vi "BRig_RT_panel_Laser1_v1,18.vi"(7 "input_setValues":bool, 9 "input_dataExp":u16[](array[numeric]), 11 "input_dataLC":u16[](array[numeric])) -> (1 "output_dataExp":u16[](array[numeric]), 3 "output_dataLC":u16[](array[numeric]))   [LabVIEW 2014]
panel:
  in  "LC_Wro_nRew2":u16
  in  "LC_Wro_nRew1":u16
  in  "LC_Rew_nRew2":u16
  in  "LC_Rew_nRew1":u16
  in  "LC_Sel_nRew2":u16
  in  "LC_Sel_nRew1":u16
  in  "LC_Cue_nRew2":u16
  in  "LC_Cue_nRew1":u16
  in  "LC_ENL_nRew2":u16
  in  "LC_ENL_nRew1":u16
  out "LaserPulseTrain":cluster{u16[], u16[]}(graph)
  in  "LED_baseline":bool
  in  "Laser_power_step":dbl
  in  "Laser_power_max":dbl
  in  "Laser_power_min":dbl
  in  "Laser_Tshutter":u16=2
  in  "Laser_Freq":u16=10
  in  "Laser_Tpeak":u16=2
  in  "Laser_T":u16
  in  "LC_Sel_PostR_Count":u16
  in  "LC_Sel_PostR_Probability":u16
  in  "LC_Sel_PostR_Block":u16(slide) max=2 step=1 scale=0.0..2.0
  in  "LC_Sel_PostR_OnOff":bool
  in  "LC_Sel_PostR_Tdelay":u16
  in  "LC_Cue_PostR_Count":u16
  in  "LC_Cue_PostR_delayOpt":bool
  in  "LC_Cue_PostR_Probability":u16
  in  "LC_Cue_PostR_Block":u16(slide) max=2 step=1 scale=0.0..2.0
  in  "LC_Cue_PostR_OnOff":bool
  in  "LC_Cue_PostR_Tdelay":u16
  in  "LC_ENL_PostR_delayOpt":bool
  in  "LC_ENL_PostR_Count":u16
  in  "LC_ENL_PostR_Probability":u16 max=100 step=1
  in  "LC_ENL_PostR_Block":u16(slide) max=2 step=1 scale=0.0..2.0
  in  "LC_ENL_PostR_OnOff":bool
  in  "LC_ENL_PostR_Tdelay":u16
  in  "LC_Sel_PreR_Count":u16
  in  "LC_Sel_First_Count":u16
  in  "LC_Sel_PreR_Probability":u16
  in  "LC_Sel_PreR_Block":u16(slide) max=2 step=1 scale=0.0..2.0
  in  "LC_Sel_PreR_OnOff":bool
  in  "LC_Sel_First_Probability":u16
  in  "LC_Sel_First_Block":u16(slide) max=2 step=1 scale=0.0..2.0
  in  "LC_Sel_First_OnOff":bool
  in  "LC_Sel_PreR_Tdelay":u16
  in  "LC_Sel_First_Tdelay":u16
  in  "LC_Cue_PreR_Count":u16
  in  "LC_Cue_First_Count":u16
  in  "LC_Cue_PreR_delayOpt":bool
  in  "LC_ENL_PreR_delayOpt":bool
  in  "LC_ENL_PreR_Count":u16
  in  "LC_ENL_First_Count":u16
  in  "LC_Cue_First_delayOpt":bool
  in  "LC_ENL_First_delayOpt":bool
  in  "LC_Wrong_Probability":u16
  in  "LC_Wrong_Trial":u16(slide) max=4 step=1 scale=0.0..4.0
  in  "LC_Wrong_Block":u16(slide) max=2 step=1 scale=0.0..2.0
  in  "LC_Wrong_OnOff":bool
  in  "LC_Reward_Probability":u16
  in  "LC_Reward_Trial":u16(slide) max=3 step=1 scale=0.0..3.0
  in  "LC_Reward_Block":u16(slide) max=2 step=1 scale=0.0..2.0
  in  "LC_Reward_OnOff":bool
  in  "LC_Cue_PreR_Probability":u16
  in  "LC_Cue_PreR_Block":u16(slide) max=2 step=1 scale=0.0..2.0
  in  "LC_Cue_PreR_OnOff":bool
  in  "LC_Cue_First_Probability":u16
  in  "LC_Cue_First_Block":u16(slide) max=2 step=1 scale=0.0..2.0
  in  "LC_Cue_First_OnOff":bool
  in  "LC_ENL_PreR_Probability":u16 max=100 step=1
  in  "LC_ENL_PreR_Block":u16(slide) max=2 step=1 scale=0.0..2.0
  in  "LC_ENL_PreR_OnOff":bool
  in  "LC_ENL_First_Probability":u16 max=100 step=1
  in  "LC_ENL_First_Block":u16(slide) max=2 step=1 scale=0.0..2.0
  in  "LC_Wrong_Tdelay":u16
  in  "LC_Cue_PreR_Tdelay":u16
  in  "LC_ENL_PreR_Tdelay":u16
  in  "LC_Reward_Tdelay":u16
  in  "LC_Cue_First_Tdelay":u16
  in  "LC_ENL_First_Tdelay":u16
  in  "LC_ENL_First_OnOff":bool
  # "Laser1 Control\n                               On/Off      Block        Probability [%]   Delay [ms]                              Count"
  # "Enforced\nNonLick"
  # "from end"
  # "First\nTrial"
  # "from start"
  # "from end"
  # "PreReward\nTrials"
  # "from start"
  # "from end"
  # "PostReward\nTrials"
  # "from start"
  # "PostReward Option - Trigger after [X1] or [X2] reward\n                                        (0 = ignore this option)"
  # "Cue"
  # "from end"
  # "First\nTrial"
  # "from start"
  # "from end"
  # "PreReward\nTrials"
  # "from start"
  # "from end"
  # "PostReward\nTrials"
  # "from start"
  # "PostReward Option - Trigger after [X1] or [X2] reward\n                                        (0 = ignore this option)"
  # "Selection"
  # "from start"
  # "First\nTrial"
  # "from start"
  # "PreReward\nTrials"
  # "from start"
  # "PostReward\nTrials"
  # "PostReward Option - Trigger after [X1] or [X2] reward\n                                        (0 = ignore this option)"
  # "Laser1 Parameters"
  # "Laser1 Response\n           On/Off      Block           Trial     Probability %  Delay [ms]"
  # "Frequency\n[Hz]"
  # "Selection\nReward"
  # "Timing [ms]\n Duration     Peak Width   Shutter"
  # "Trigger after [X1] or [X2] reward\n(0 = ignore this option)"
  # "Laser Power [V]\nMin          Max              Step"
  # "Selection\nWrong"
  # "Trigger after [X1] or [X2] reward\n(0 = ignore this option)"
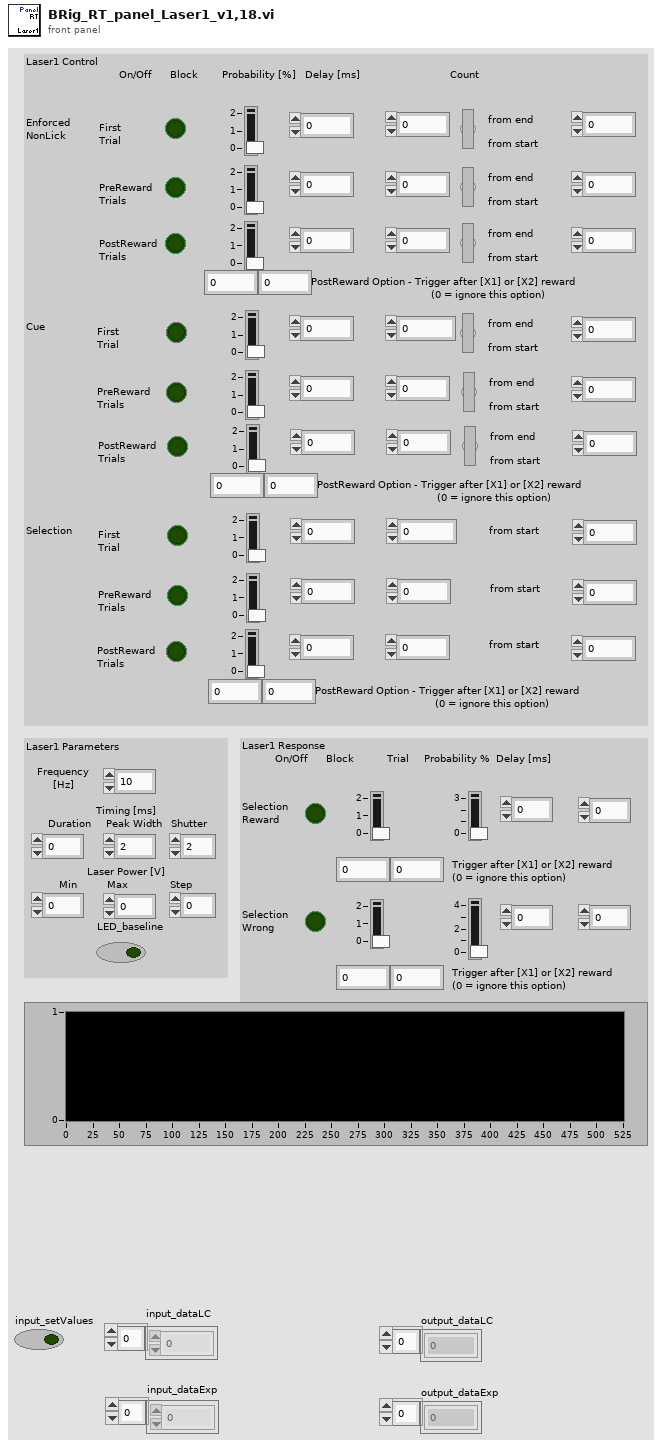
[diagram p1: front panel]
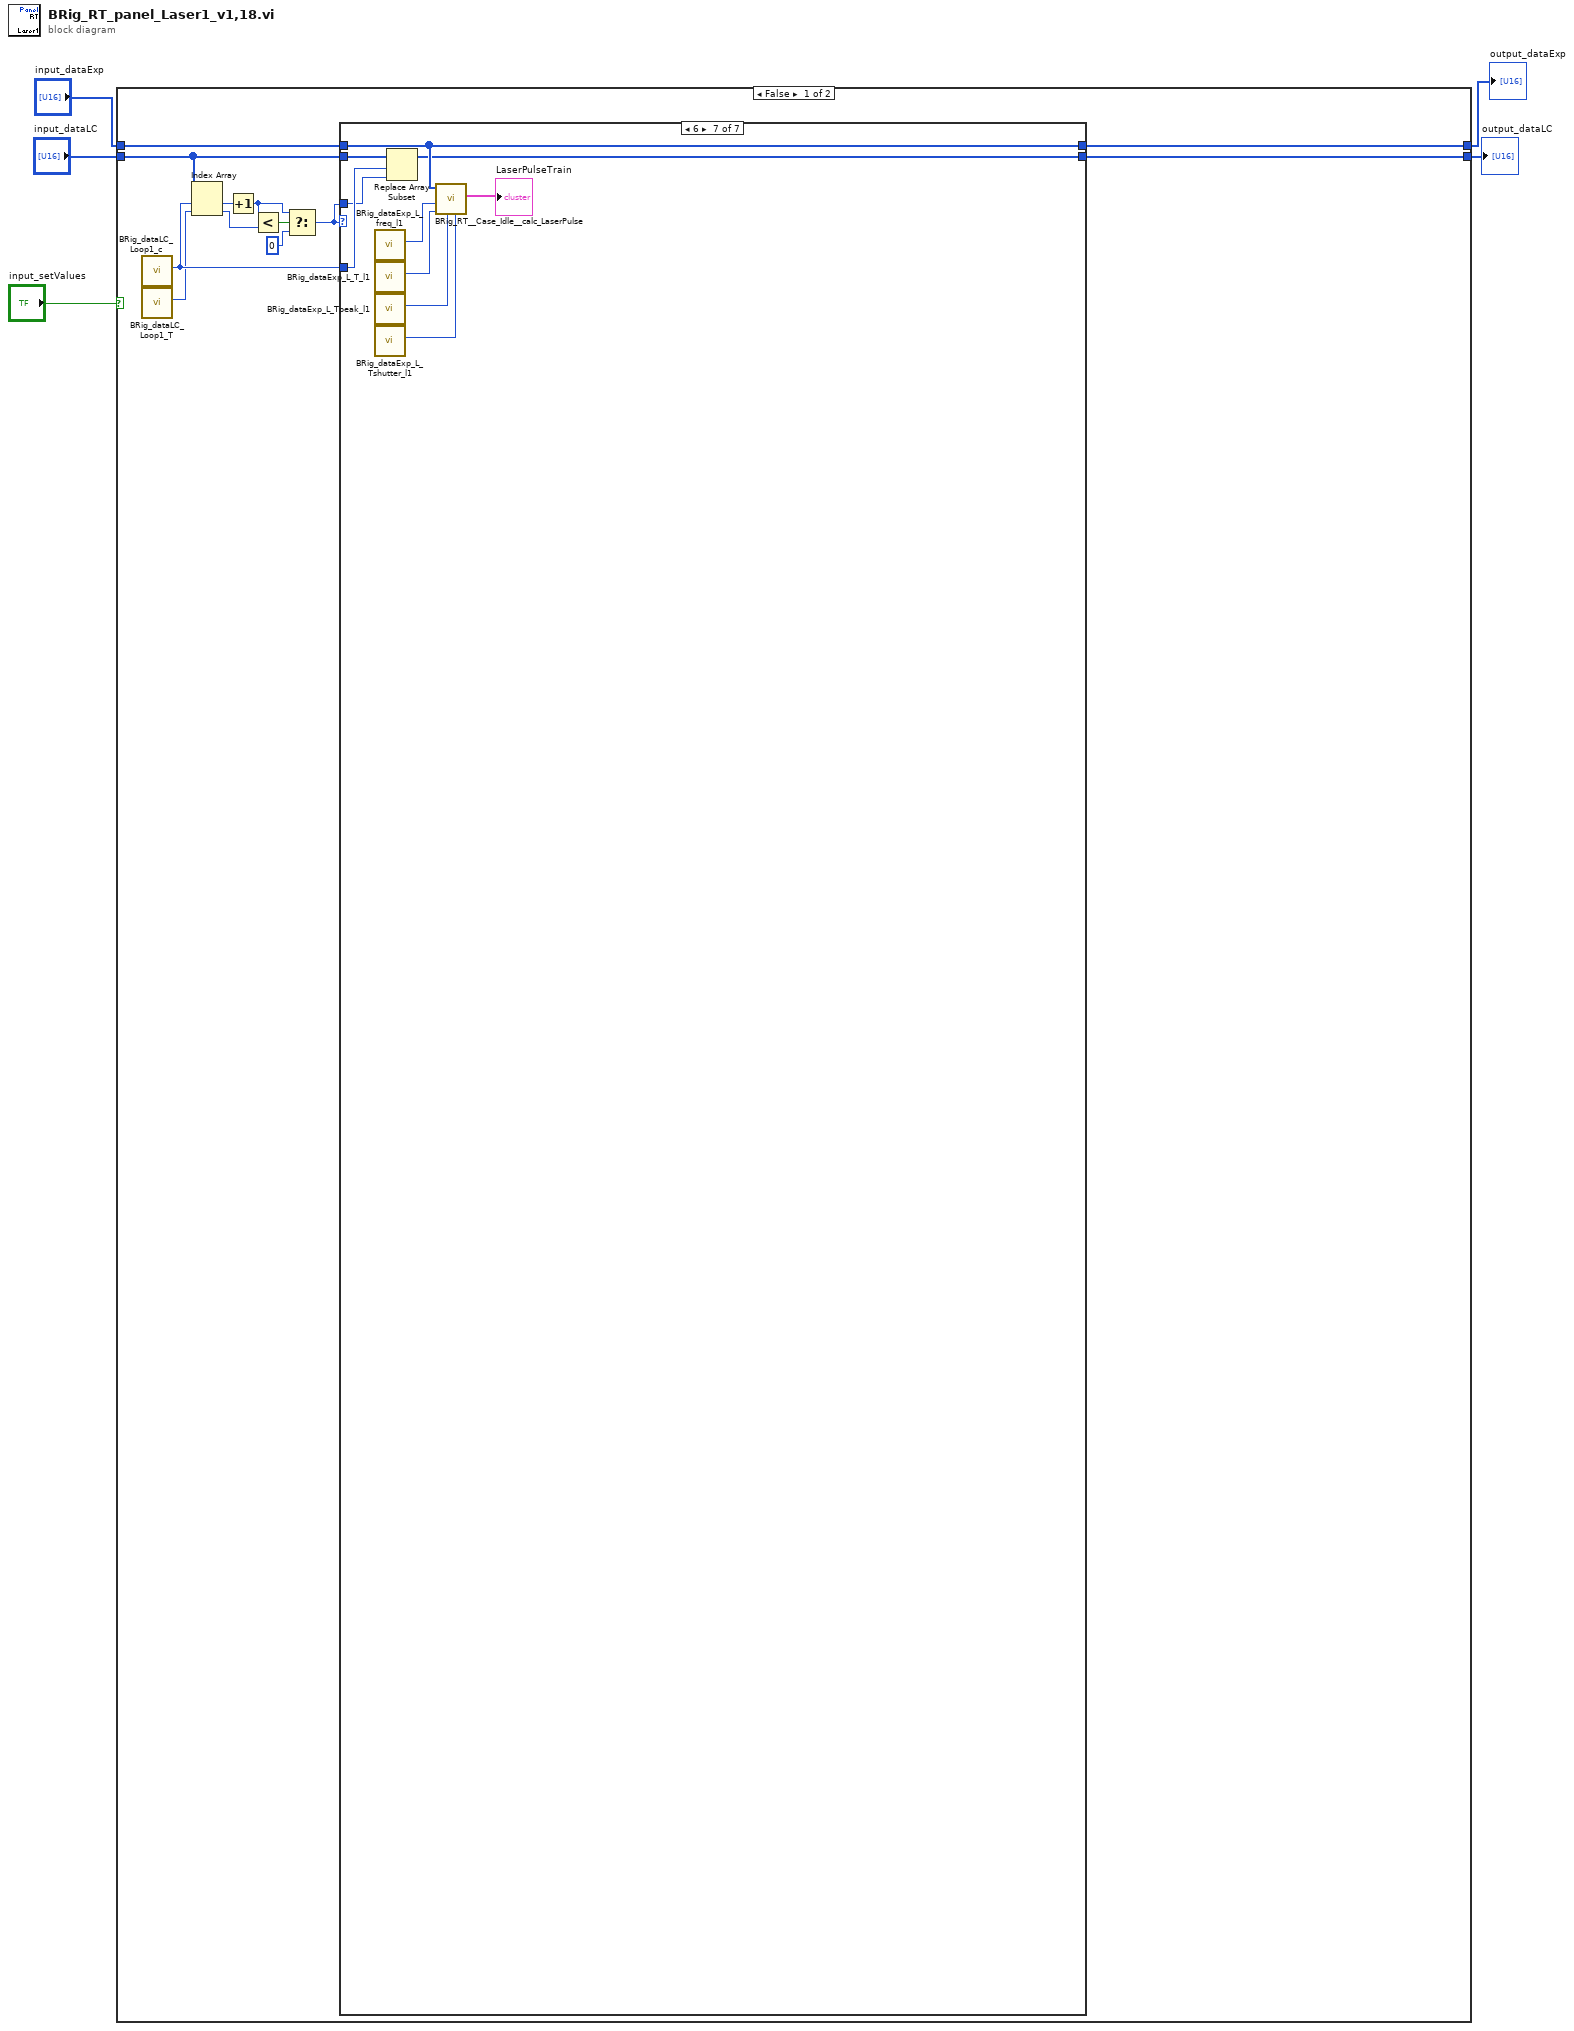
[diagram p0: block diagram]
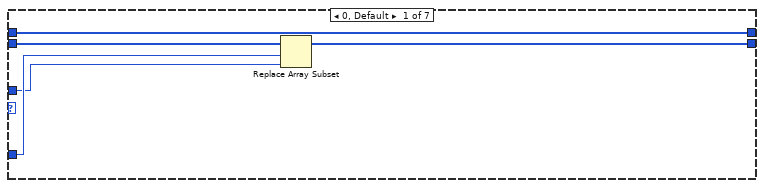
[diagram p2: hidden frame]
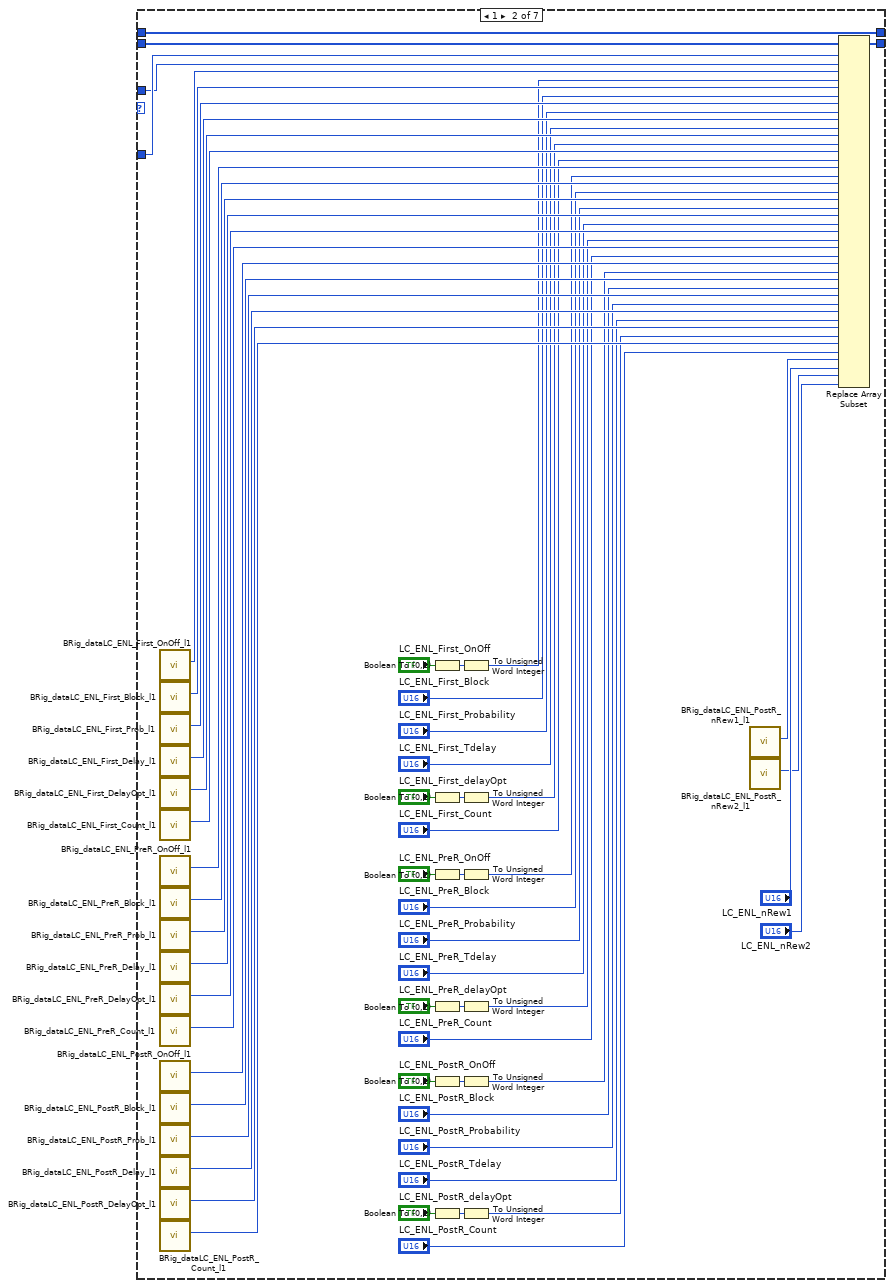
[diagram p3: hidden frame]
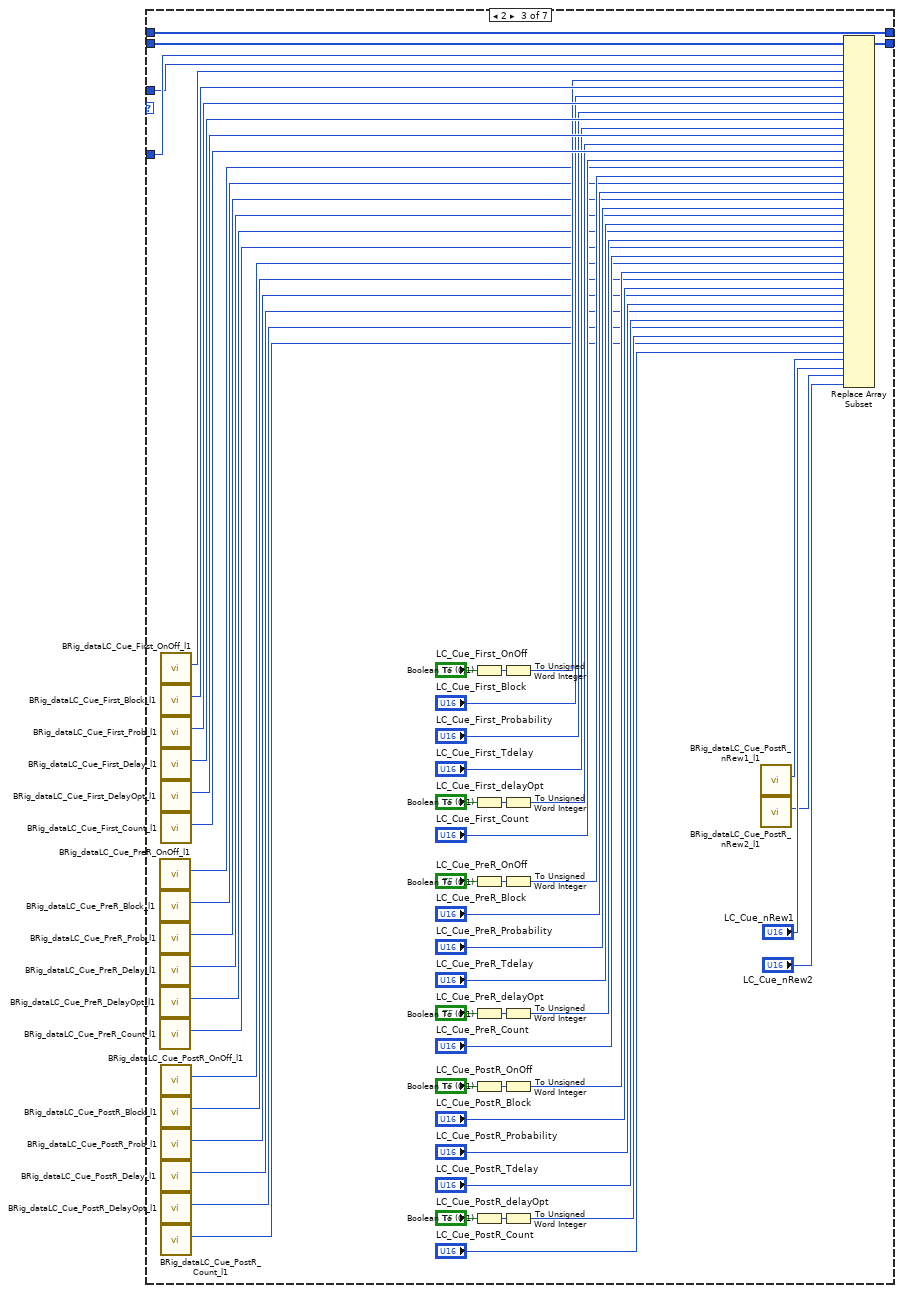
[diagram p4: hidden frame]
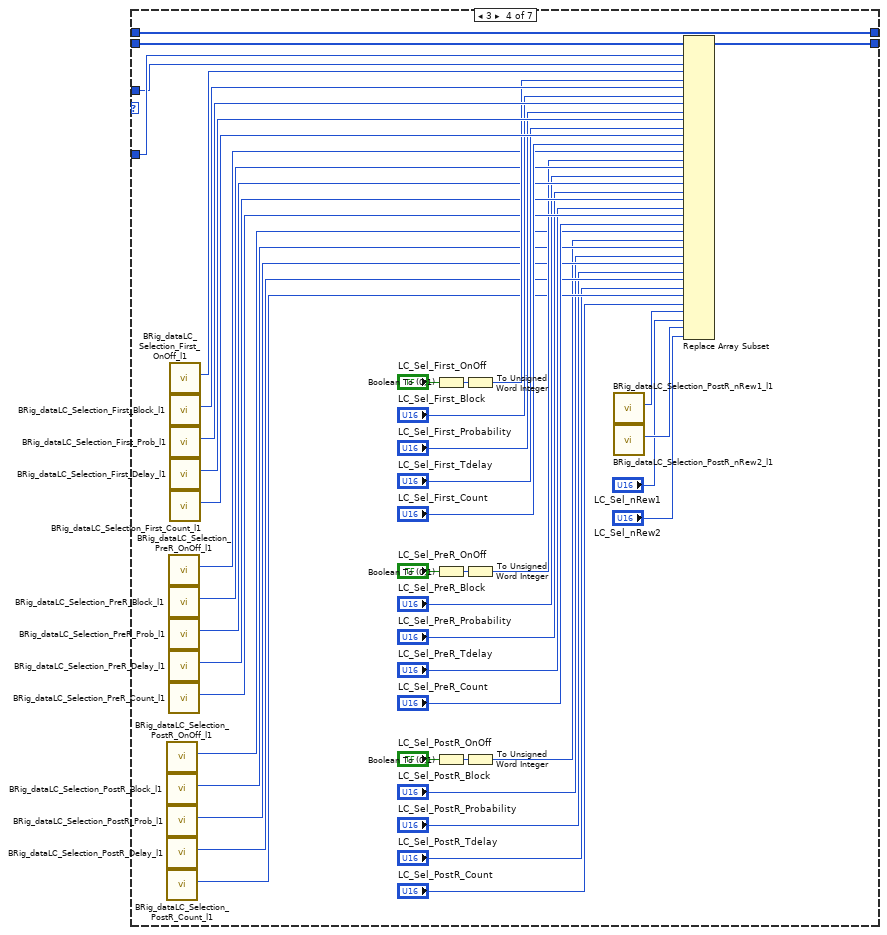
[diagram p5: hidden frame]
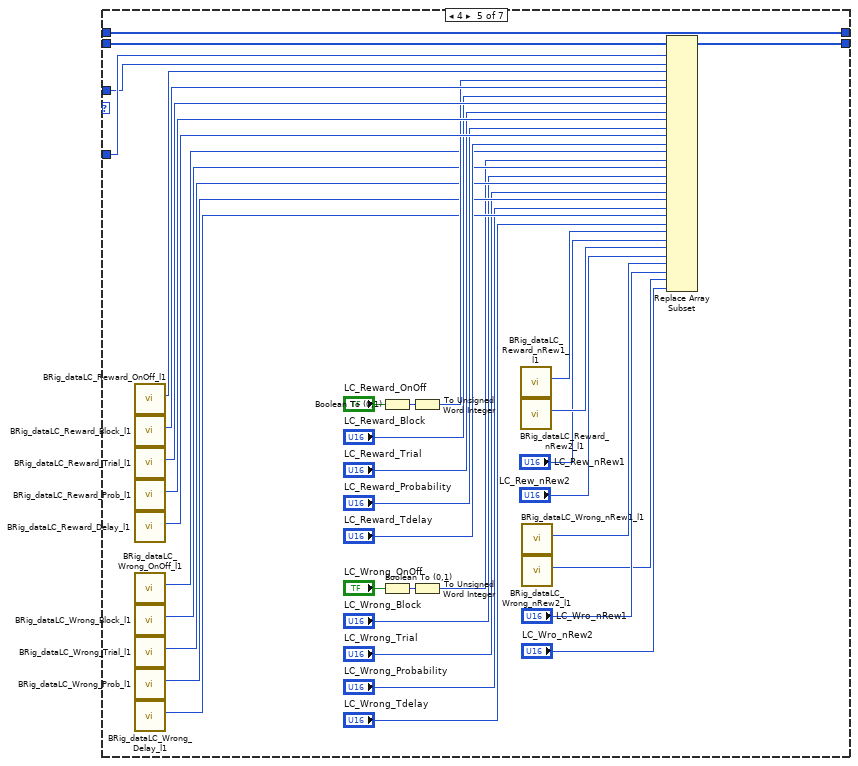
[diagram p6: hidden frame]
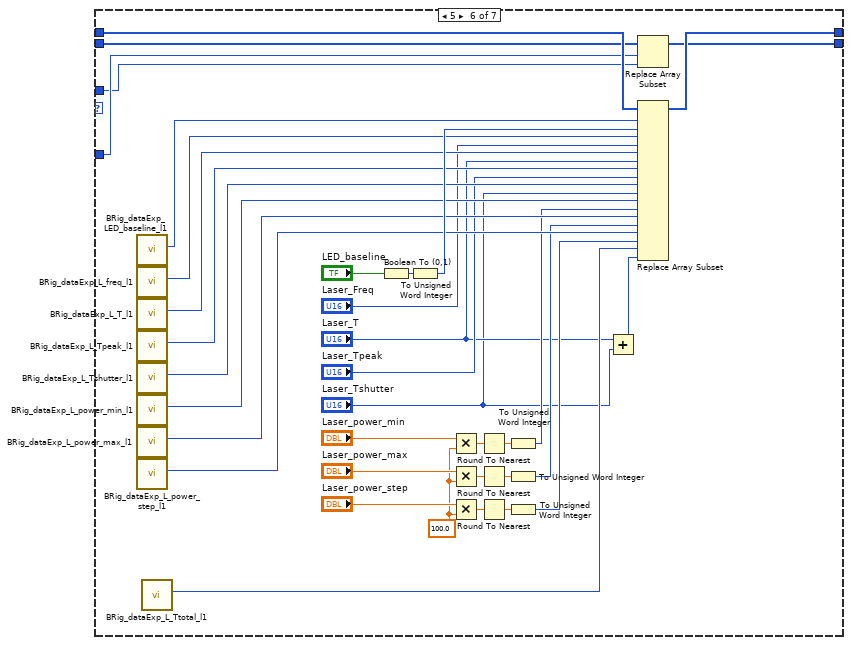
[diagram p7: hidden frame]
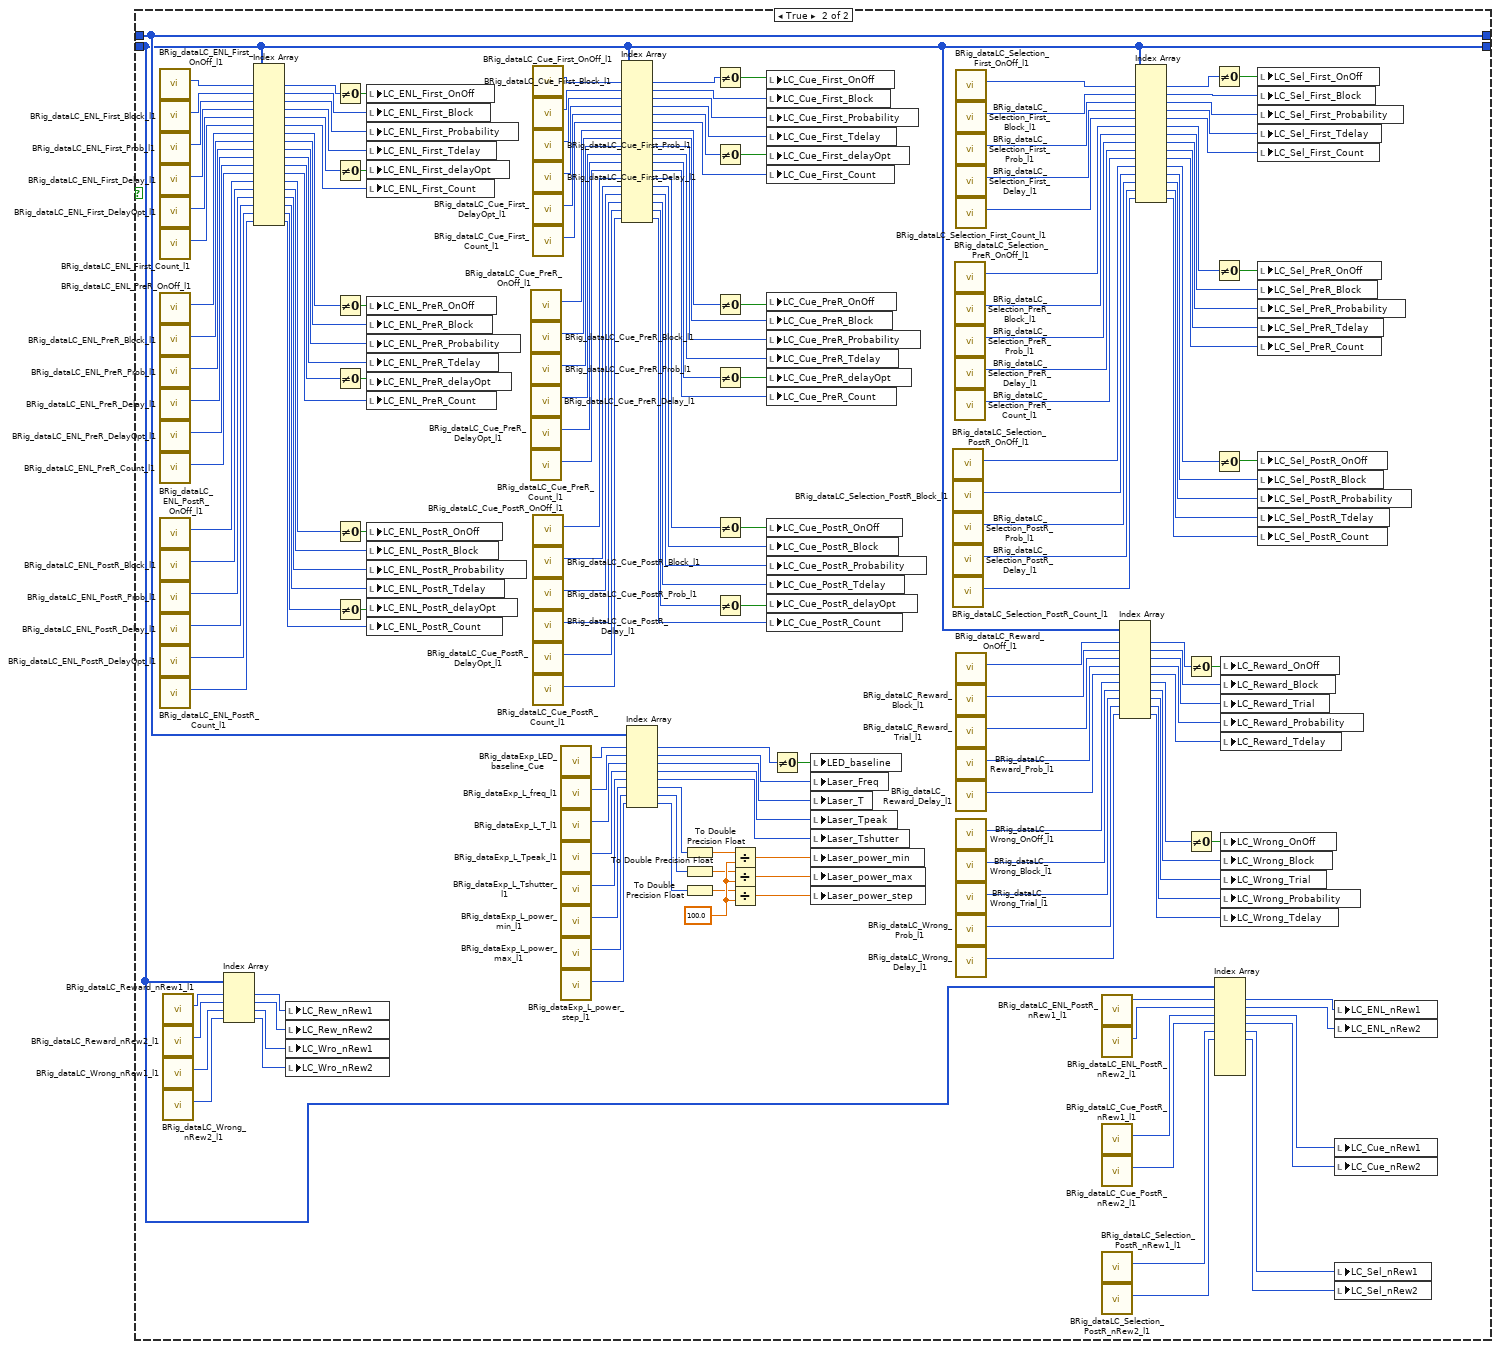
[diagram p8: hidden frame]
diagram:
  n1 = case shown="False" "input_setValues" {
    tunnel: "input_dataLC" -> [w17 w281]
    tunnel: [w11 w281] -> w4
    tunnel: "input_dataExp" -> [w7 w282]
    tunnel: [w6 w282] -> w1
    frame False {
      n2 = call "BRig_dataLC_Loop1_c.vi"() -> ("output_Loop1_c"=w10:i32)  [unwired: 11 in]
      n3 = call "BRig_dataLC_Loop1_T.vi"() -> ("output_Loop1_T"=w9:i32)  [unwired: 11 in]
      n4 = Index Array(array=w17, index #1=w10, index #2=w9) -> (element #1=w16:u16, element #2=w15:u16)
      n5 = Increment(x=w16) -> (x+1=w12:u16)
      n6 = Less?(x=w12, y=w15) -> (x < y?=w14:bool)
      n7 = Select(t=w12, s=w14, f=u16 0) -> (s? t:f=w8:u16)
      n8 = case shown="6" w8 {
        tunnel: w17 -> [w22 w79 w136 w181 w218 w223 w262]
        tunnel: w10 -> [w20 w29 w98 w143 w192 w221 w260]
        tunnel: w8 -> [w19 w28 w97 w142 w191 w220 w259]
        tunnel: [w21 w72 w135 w180 w217 w222 w261] -> w11
        tunnel: w7 -> [w18 w27 w84 w141 w190 w225 w264]
        tunnel: [w18 w27 w84 w141 w190 w224 w264] -> w6
        frame 0, Default {
          n9 = Replace Array Subset(array=w22, new element=w19, index=w20) -> (w21:u16[])
        }
        frame 1 {
          n10 = call "BRig_dataLC_ENL_First_OnOff_l1.vi"() -> ("output_ENL_First_OnOff"=w78:i32)  [unwired: 11 in]
          n11 = call "BRig_dataLC_ENL_First_Block_l1.vi"() -> ("output_ENL_First_Block"=w77:i32)  [unwired: 11 in]
          n12 = call "BRig_dataLC_ENL_First_Prob_l1.vi"() -> ("output_ENL_First_Prob"=w76:i32)  [unwired: 11 in]
          n13 = call "BRig_dataLC_ENL_First_Delay_l1.vi"() -> ("output_ENL_First_Delay"=w75:i32)  [unwired: 11 in]
          n14 = call "BRig_dataLC_ENL_First_DelayOpt_l1.vi"() -> ("output_ENL_First_DelayOpt"=w74:i32)  [unwired: 11 in]
          n15 = call "BRig_dataLC_ENL_First_Count_l1.vi"() -> ("output_ENL_First_Count"=w73:i32)  [unwired: 11 in]
          n16 = call "BRig_dataLC_ENL_PreR_OnOff_l1.vi"() -> ("output_ENL_PreR_OnOff"=w71:i32)  [unwired: 11 in]
          n17 = call "BRig_dataLC_ENL_PreR_Block_l1.vi"() -> ("output_ENL_PreR_Block"=w70:i32)  [unwired: 11 in]
          n18 = call "BRig_dataLC_ENL_PreR_Prob_l1.vi"() -> ("output_ENL_PreR_Prob"=w69:i32)  [unwired: 11 in]
          n19 = call "BRig_dataLC_ENL_PreR_Delay_l1.vi"() -> ("output_ENL_PreR_Delay"=w68:i32)  [unwired: 11 in]
          n20 = call "BRig_dataLC_ENL_PreR_DelayOpt_l1.vi"() -> ("output_ENL_PreR_DelayOpt"=w67:i32)  [unwired: 11 in]
          n21 = call "BRig_dataLC_ENL_PreR_Count_l1.vi"() -> ("output_ENL_PreR_Count"=w66:i32)  [unwired: 11 in]
          n22 = call "BRig_dataLC_ENL_PostR_OnOff_l1.vi"() -> ("output_ENL_PostR_OnOff"=w65:i32)  [unwired: 11 in]
          n23 = call "BRig_dataLC_ENL_PostR_Block_l1.vi"() -> ("output_ENL_PostR_Block"=w64:i32)  [unwired: 11 in]
          n24 = call "BRig_dataLC_ENL_PostR_Prob_l1.vi"() -> ("output_ENL_PostR_Prob"=w63:i32)  [unwired: 11 in]
          n25 = call "BRig_dataLC_ENL_PostR_Delay_l1.vi"() -> ("output_ENL_PostR_Delay"=w62:i32)  [unwired: 11 in]
          n26 = call "BRig_dataLC_ENL_PostR_DelayOpt_l1.vi"() -> ("output_ENL_PostR_DelayOpt"=w61:i32)  [unwired: 11 in]
          n27 = call "BRig_dataLC_ENL_PostR_Count_l1.vi"() -> ("output_ENL_PostR_Count"=w60:i32)  [unwired: 11 in]
          n28 = Boolean To (0,1)(Boolean="LC_ENL_First_OnOff") -> (0, 1=w58:i16)
          n29 = Boolean To (0,1)(Boolean="LC_ENL_First_delayOpt") -> (0, 1=w57:i16)
          n30 = Boolean To (0,1)(Boolean="LC_ENL_PreR_OnOff") -> (0, 1=w55:i16)
          n31 = Boolean To (0,1)(Boolean="LC_ENL_PreR_delayOpt") -> (0, 1=w53:i16)
          n32 = Boolean To (0,1)(Boolean="LC_ENL_PostR_OnOff") -> (0, 1=w51:i16)
          n33 = Boolean To (0,1)(Boolean="LC_ENL_PostR_delayOpt") -> (0, 1=w49:i16)
          n34 = To Unsigned Word Integer(number=w58) -> (unsigned 16bit integer=w47:u16)
          n35 = To Unsigned Word Integer(number=w57) -> (unsigned 16bit integer=w43:u16)
          n36 = To Unsigned Word Integer(number=w55) -> (unsigned 16bit integer=w41:u16)
          n37 = To Unsigned Word Integer(number=w53) -> (unsigned 16bit integer=w37:u16)
          n38 = To Unsigned Word Integer(number=w51) -> (unsigned 16bit integer=w35:u16)
          n39 = To Unsigned Word Integer(number=w49) -> (unsigned 16bit integer=w31:u16)
          n40 = call "BRig_dataLC_ENL_PostR_nRew1_l1.vi"() -> ("output_ENL_PostR_nRew1_l1"=w26:i32)  [unwired: 11 in]
          n41 = call "BRig_dataLC_ENL_PostR_nRew2_l1.vi"() -> ("output_ENL_PostR_nRew2_l1"=w24:i32)  [unwired: 11 in]
          n42 = Replace Array Subset(array=w79, new element #1=w28, index #1=w29, new element #2=w47, index #2=w78, new element #3="LC_ENL_First_Block", index #3=w77, new element #4="LC_ENL_First_Probability", index #4=w76, new element #5="LC_ENL_First_Tdelay", index #5=w75, new element #6=w43, index #6=w74, new element #7="LC_ENL_First_Count", index #7=w73, new element #8=w41, index #8=w71, new element #9="LC_ENL_PreR_Block", index #9=w70, new element #10="LC_ENL_PreR_Probability", index #10=w69, new element #11="LC_ENL_PreR_Tdelay", index #11=w68, new element #12=w37, index #12=w67, new element #13="LC_ENL_PreR_Count", index #13=w66, new element #14=w35, index #14=w65, new element #15="LC_ENL_PostR_Block", index #15=w64, new element #16="LC_ENL_PostR_Probability", index #16=w63, new element #17="LC_ENL_PostR_Tdelay", index #17=w62, new element #18=w31, index #18=w61, new element #19="LC_ENL_PostR_Count", index #19=w60, new element #20="LC_ENL_nRew1", index #20=w26, new element #21="LC_ENL_nRew2", index #21=w24) -> (w72:u16[])
        }
        frame 2 {
          n43 = call "BRig_dataLC_Cue_PreR_OnOff_l1.vi"() -> ("output_Cue_PreR_OnOff"=w94:i32)  [unwired: 11 in]
          n44 = call "BRig_dataLC_Cue_PreR_Block_l1.vi"() -> ("output_Cue_PreR_Block"=w93:i32)  [unwired: 11 in]
          n45 = call "BRig_dataLC_Cue_PreR_Prob_l1.vi"() -> ("output_Cue_PreR_Prob"=w92:i32)  [unwired: 11 in]
          n46 = call "BRig_dataLC_Cue_PreR_Delay_l1.vi"() -> ("output_Cue_PreR_Delay"=w91:i32)  [unwired: 11 in]
          n47 = call "BRig_dataLC_Cue_PreR_DelayOpt_l1.vi"() -> ("output_Cue_PreR_DelayOpt"=w90:i32)  [unwired: 11 in]
          n48 = call "BRig_dataLC_Cue_PreR_Count_l1.vi"() -> ("output_Cue_PreR_Count"=w95:i32)  [unwired: 11 in]
          n49 = call "BRig_dataLC_Cue_First_OnOff_l1.vi"() -> ("output_Cue_First_OnOff"=w134:i32)  [unwired: 11 in]
          n50 = call "BRig_dataLC_Cue_First_Block_l1.vi"() -> ("output_Cue_First_Block"=w133:i32)  [unwired: 11 in]
          n51 = call "BRig_dataLC_Cue_First_Prob_l1.vi"() -> ("output_Cue_First_Prob"=w132:i32)  [unwired: 11 in]
          n52 = call "BRig_dataLC_Cue_First_Delay_l1.vi"() -> ("output_Cue_First_Delay"=w131:i32)  [unwired: 11 in]
          n53 = call "BRig_dataLC_Cue_First_DelayOpt_l1.vi"() -> ("output_Cue_First_DelayOpt"=w130:i32)  [unwired: 11 in]
          n54 = call "BRig_dataLC_Cue_First_Count_l1.vi"() -> ("output_Cue_First_Count"=w129:i32)  [unwired: 11 in]
          n55 = call "BRig_dataLC_Cue_PostR_OnOff_l1.vi"() -> ("output_Cue_PostR_OnOff"=w96:i32)  [unwired: 11 in]
          n56 = call "BRig_dataLC_Cue_PostR_Block_l1.vi"() -> ("output_Cue_PostR_Block"=w89:i32)  [unwired: 11 in]
          n57 = call "BRig_dataLC_Cue_PostR_Prob_l1.vi"() -> ("output_Cue_PostR_Prob"=w88:i32)  [unwired: 11 in]
          n58 = call "BRig_dataLC_Cue_PostR_Delay_l1.vi"() -> ("output_Cue_PostR_Delay"=w87:i32)  [unwired: 11 in]
          n59 = call "BRig_dataLC_Cue_PostR_DelayOpt_l1.vi"() -> ("output_Cue_PostR_DelayOpt"=w86:i32)  [unwired: 11 in]
          n60 = call "BRig_dataLC_Cue_PostR_Count_l1.vi"() -> ("output_Cue_PostR_Count"=w85:i32)  [unwired: 11 in]
          n61 = Boolean To (0,1)(Boolean="LC_Cue_First_OnOff") -> (0, 1=w122:i16)
          n62 = Boolean To (0,1)(Boolean="LC_Cue_First_delayOpt") -> (0, 1=w121:i16)
          n63 = Boolean To (0,1)(Boolean="LC_Cue_PreR_OnOff") -> (0, 1=w120:i16)
          n64 = Boolean To (0,1)(Boolean="LC_Cue_PreR_delayOpt") -> (0, 1=w119:i16)
          n65 = Boolean To (0,1)(Boolean="LC_Cue_PostR_OnOff") -> (0, 1=w118:i16)
          n66 = Boolean To (0,1)(Boolean="LC_Cue_PostR_delayOpt") -> (0, 1=w117:i16)
          n67 = To Unsigned Word Integer(number=w122) -> (unsigned 16bit integer=w116:u16)
          n68 = To Unsigned Word Integer(number=w121) -> (unsigned 16bit integer=w112:u16)
          n69 = To Unsigned Word Integer(number=w120) -> (unsigned 16bit integer=w110:u16)
          n70 = To Unsigned Word Integer(number=w119) -> (unsigned 16bit integer=w106:u16)
          n71 = To Unsigned Word Integer(number=w118) -> (unsigned 16bit integer=w104:u16)
          n72 = To Unsigned Word Integer(number=w117) -> (unsigned 16bit integer=w100:u16)
          n73 = call "BRig_dataLC_Cue_PostR_nRew1_l1.vi"() -> ("output_Cue_PostR_nRew1_l1"=w83:i32)  [unwired: 11 in]
          n74 = call "BRig_dataLC_Cue_PostR_nRew2_l1.vi"() -> ("output_Cue_PostR_nRew2_l1"=w81:i32)  [unwired: 11 in]
          n75 = Replace Array Subset(array=w136, new element #1=w97, index #1=w98, new element #2=w116, index #2=w134, new element #3="LC_Cue_First_Block", index #3=w133, new element #4="LC_Cue_First_Probability", index #4=w132, new element #5="LC_Cue_First_Tdelay", index #5=w131, new element #6=w112, index #6=w130, new element #7="LC_Cue_First_Count", index #7=w129, new element #8=w110, index #8=w94, new element #9="LC_Cue_PreR_Block", index #9=w93, new element #10="LC_Cue_PreR_Probability", index #10=w92, new element #11="LC_Cue_PreR_Tdelay", index #11=w91, new element #12=w106, index #12=w90, new element #13="LC_Cue_PreR_Count", index #13=w95, new element #14=w104, index #14=w96, new element #15="LC_Cue_PostR_Block", index #15=w89, new element #16="LC_Cue_PostR_Probability", index #16=w88, new element #17="LC_Cue_PostR_Tdelay", index #17=w87, new element #18=w100, index #18=w86, new element #19="LC_Cue_PostR_Count", index #19=w85, new element #20="LC_Cue_nRew1", index #20=w83, new element #21="LC_Cue_nRew2", index #21=w81) -> (w135:u16[])
        }
        frame 3 {
          n76 = call "BRig_dataLC_Selection_PostR_OnOff_l1.vi"() -> ("output_Selection_PostR_OnOff"=w153:i32)  [unwired: 11 in]
          n77 = call "BRig_dataLC_Selection_PostR_Block_l1.vi"() -> ("output_Selection_PostR_Block"=w152:i32)  [unwired: 11 in]
          n78 = call "BRig_dataLC_Selection_PostR_Prob_l1.vi"() -> ("output_Selection_PostR_Prob"=w151:i32)  [unwired: 11 in]
          n79 = call "BRig_dataLC_Selection_PostR_Delay_l1.vi"() -> ("output_Selection_PostR_Delay"=w150:i32)  [unwired: 11 in]
          n80 = call "BRig_dataLC_Selection_PostR_Count_l1.vi"() -> ("output_Selection_PostR_Count"=w149:i32)  [unwired: 11 in]
          n81 = call "BRig_dataLC_Selection_PreR_OnOff_l1.vi"() -> ("output_Selection_PreR_OnOff"=w163:i32)  [unwired: 11 in]
          n82 = call "BRig_dataLC_Selection_PreR_Block_l1.vi"() -> ("output_Selection_PreR_Block"=w162:i32)  [unwired: 11 in]
          n83 = call "BRig_dataLC_Selection_PreR_Prob_l1.vi"() -> ("output_Selection_PreR_Prob"=w161:i32)  [unwired: 11 in]
          n84 = call "BRig_dataLC_Selection_PreR_Delay_l1.vi"() -> ("output_Selection_PreR_Delay"=w160:i32)  [unwired: 11 in]
          n85 = call "BRig_dataLC_Selection_PreR_Count_l1.vi"() -> ("output_Selection_PreR_Count"=w159:i32)  [unwired: 11 in]
          n86 = call "BRig_dataLC_Selection_First_OnOff_l1.vi"() -> ("output_Selection_First_OnOff"=w173:i32)  [unwired: 11 in]
          n87 = call "BRig_dataLC_Selection_First_Block_l1.vi"() -> ("output_Selection_First_Block"=w172:i32)  [unwired: 11 in]
          n88 = call "BRig_dataLC_Selection_First_Prob_l1.vi"() -> ("output_Selection_First_Prob"=w171:i32)  [unwired: 11 in]
          n89 = call "BRig_dataLC_Selection_First_Delay_l1.vi"() -> ("output_Selection_First_Delay"=w170:i32)  [unwired: 11 in]
          n90 = call "BRig_dataLC_Selection_First_Count_l1.vi"() -> ("output_Selection_First_Count"=w169:i32)  [unwired: 11 in]
          n91 = Boolean To (0,1)(Boolean="LC_Sel_First_OnOff") -> (0, 1=w176:i16)
          n92 = Boolean To (0,1)(Boolean="LC_Sel_PreR_OnOff") -> (0, 1=w175:i16)
          n93 = Boolean To (0,1)(Boolean="LC_Sel_PostR_OnOff") -> (0, 1=w174:i16)
          n94 = To Unsigned Word Integer(number=w176) -> (unsigned 16bit integer=w168:u16)
          n95 = To Unsigned Word Integer(number=w175) -> (unsigned 16bit integer=w158:u16)
          n96 = To Unsigned Word Integer(number=w174) -> (unsigned 16bit integer=w148:u16)
          n97 = call "BRig_dataLC_Selection_PostR_nRew1_l1.vi"() -> ("output_Selection_PostR_nRew1_l1"=w140:i32)  [unwired: 11 in]
          n98 = call "BRig_dataLC_Selection_PostR_nRew2_l1.vi"() -> ("output_Selection_PostR_nRew2_l1"=w139:i32)  [unwired: 11 in]
          n99 = Replace Array Subset(array=w181, new element #1=w142, index #1=w143, new element #2=w168, index #2=w173, new element #3="LC_Sel_First_Block", index #3=w172, new element #4="LC_Sel_First_Probability", index #4=w171, new element #5="LC_Sel_First_Tdelay", index #5=w170, new element #6="LC_Sel_First_Count", index #6=w169, new element #7=w158, index #7=w163, new element #8="LC_Sel_PreR_Block", index #8=w162, new element #9="LC_Sel_PreR_Probability", index #9=w161, new element #10="LC_Sel_PreR_Tdelay", index #10=w160, new element #11="LC_Sel_PreR_Count", index #11=w159, new element #12=w148, index #12=w153, new element #13="LC_Sel_PostR_Block", index #13=w152, new element #14="LC_Sel_PostR_Probability", index #14=w151, new element #15="LC_Sel_PostR_Tdelay", index #15=w150, new element #16="LC_Sel_PostR_Count", index #16=w149, new element #17="LC_Sel_nRew1", index #17=w140, new element #18="LC_Sel_nRew2", index #18=w139) -> (w180:u16[])
        }
        frame 4 {
          n100 = call "BRig_dataLC_Reward_OnOff_l1.vi"() -> ("output_Reward_OnOff"=w216:i32)  [unwired: 11 in]
          n101 = call "BRig_dataLC_Reward_Block_l1.vi"() -> ("output_Reward_Block"=w215:i32)  [unwired: 11 in]
          n102 = call "BRig_dataLC_Reward_Trial_l1.vi"() -> ("output_Reward_Trial"=w214:i32)  [unwired: 11 in]
          n103 = call "BRig_dataLC_Reward_Prob_l1.vi"() -> ("output_Reward_Prob"=w213:i32)  [unwired: 11 in]
          n104 = call "BRig_dataLC_Reward_Delay_l1.vi"() -> ("output_Reward_Delay"=w212:i32)  [unwired: 11 in]
          n105 = call "BRig_dataLC_Wrong_OnOff_l1.vi"() -> ("output_Wrong_OnOff"=w202:i32)  [unwired: 11 in]
          n106 = call "BRig_dataLC_Wrong_Block_l1.vi"() -> ("output_Wrong_Block"=w201:i32)  [unwired: 11 in]
          n107 = call "BRig_dataLC_Wrong_Trial_l1.vi"() -> ("output_Wrong_Trial"=w200:i32)  [unwired: 11 in]
          n108 = call "BRig_dataLC_Wrong_Prob_l1.vi"() -> ("output_Wrong_Prob"=w199:i32)  [unwired: 11 in]
          n109 = call "BRig_dataLC_Wrong_Delay_l1.vi"() -> ("output_Wrong_Delay"=w198:i32)  [unwired: 11 in]
          n110 = Boolean To (0,1)(Boolean="LC_Reward_OnOff") -> (0, 1=w209:i16)
          n111 = Boolean To (0,1)(Boolean="LC_Wrong_OnOff") -> (0, 1=w208:i16)
          n112 = To Unsigned Word Integer(number=w209) -> (unsigned 16bit integer=w207:u16)
          n113 = To Unsigned Word Integer(number=w208) -> (unsigned 16bit integer=w197:u16)
          n114 = call "BRig_dataLC_Reward_nRew1_l1.vi"() -> ("output_Reward_nRew1_l1"=w189:i32)  [unwired: 11 in]
          n115 = call "BRig_dataLC_Reward_nRew2_l1.vi"() -> ("output_Reward_nRew2_l1"=w188:i32)  [unwired: 11 in]
          n116 = call "BRig_dataLC_Wrong_nRew1_l1.vi"() -> ("output_Wrong_nRew1_l1"=w185:i32)  [unwired: 11 in]
          n117 = call "BRig_dataLC_Wrong_nRew2_l1.vi"() -> ("output_Wrong_nRew2_l1"=w183:i32)  [unwired: 11 in]
          n118 = Replace Array Subset(array=w218, new element #1=w191, index #1=w192, new element #2=w207, index #2=w216, new element #3="LC_Reward_Block", index #3=w215, new element #4="LC_Reward_Trial", index #4=w214, new element #5="LC_Reward_Probability", index #5=w213, new element #6="LC_Reward_Tdelay", index #6=w212, new element #7=w197, index #7=w202, new element #8="LC_Wrong_Block", index #8=w201, new element #9="LC_Wrong_Trial", index #9=w200, new element #10="LC_Wrong_Probability", index #10=w199, new element #11="LC_Wrong_Tdelay", index #11=w198, new element #12="LC_Rew_nRew1", index #12=w189, new element #13="LC_Rew_nRew2", index #13=w188, new element #14="LC_Wro_nRew1", index #14=w185, new element #15="LC_Wro_nRew2", index #15=w183) -> (w217:u16[])
        }
        frame 5 {
          w242 = 100.0 ("y")
          n119 = call "BRig_dataExp_LED_baseline_l1.vi"() -> ("output_LED_baseline_l1"=w219:i32)  [unwired: 11 in]
          n120 = call "BRig_dataExp_L_freq_l1.vi"() -> ("output_L_freq_l1"=w241:i32)  [unwired: 11 in]
          n121 = call "BRig_dataExp_L_T_l1.vi"() -> ("output_L_T_l1"=w240:i32)  [unwired: 11 in]
          n122 = call "BRig_dataExp_L_Tpeak_l1.vi"() -> ("output_L_Tpeak_l1"=w239:i32)  [unwired: 11 in]
          n123 = call "BRig_dataExp_L_Tshutter_l1.vi"() -> ("output_L_Tshutter_l1"=w238:i32)  [unwired: 11 in]
          n124 = call "BRig_dataExp_L_power_min_l1.vi"() -> ("output_L_power_min_l1"=w237:i32)  [unwired: 11 in]
          n125 = call "BRig_dataExp_L_power_max_l1.vi"() -> ("output_L_power_max_l1"=w236:i32)  [unwired: 11 in]
          n126 = call "BRig_dataExp_L_power_step_l1.vi"() -> ("output_L_power_step_l1"=w235:i32)  [unwired: 11 in]
          n127 = call "BRig_dataExp_L_Ttotal_l1.vi"() -> ("output_L_Ttotal_l1"=w229:i32)  [unwired: 11 in]
          n128 = Boolean To (0,1)(Boolean="LED_baseline") -> (0, 1=w254:i16)
          n129 = To Unsigned Word Integer(number=w254) -> (unsigned 16bit integer=w252:u16)
          n130 = Multiply(x="Laser_power_min", y=w242) -> (x*y=w246:dbl)
          n131 = Multiply(x="Laser_power_max", y=w242) -> (x*y=w248:dbl)
          n132 = Multiply(x="Laser_power_step", y=w242) -> (x*y=w251:dbl)
          n133 = Round To Nearest(number=w246) -> (nearest integer value=w245:dbl)
          n134 = Round To Nearest(number=w248) -> (nearest integer value=w247:dbl)
          n135 = Round To Nearest(number=w251) -> (nearest integer value=w250:dbl)
          n136 = To Unsigned Word Integer(number=w245) -> (unsigned 16bit integer=w232:u16)
          n137 = To Unsigned Word Integer(number=w247) -> (unsigned 16bit integer=w233:u16)
          n138 = To Unsigned Word Integer(number=w250) -> (unsigned 16bit integer=w234:u16)
          n139 = Add(x="Laser_T", y="Laser_Tshutter") -> (x+y=w226:u16)
          n140 = Replace Array Subset(array=w223, new element=w220, index=w221) -> (w222:u16[])
          n141 = Replace Array Subset(array=w225, new element #1=w252, index #1=w219, new element #2="Laser_Freq", index #2=w241, new element #3="Laser_T", index #3=w240, new element #4="Laser_Tpeak", index #4=w239, new element #5="Laser_Tshutter", index #5=w238, new element #6=w232, index #6=w237, new element #7=w233, index #7=w236, new element #8=w234, index #8=w235, new element #9=w226, index #9=w229) -> (w224:u16[])
        }
        frame 6 {
          n142 = call "BRig_dataExp_L_freq_l1.vi"() -> ("output_L_freq_l1"=w257:i32)  [unwired: 11 in]
          n143 = call "BRig_dataExp_L_T_l1.vi"() -> ("output_L_T_l1"=w258:i32)  [unwired: 11 in]
          n144 = call "BRig_dataExp_L_Tpeak_l1.vi"() -> ("output_L_Tpeak_l1"=w256:i32)  [unwired: 11 in]
          n145 = call "BRig_dataExp_L_Tshutter_l1.vi"() -> ("output_L_Tshutter_l1"=w255:i32)  [unwired: 11 in]
          n146 = Replace Array Subset(array=w262, new element=w259, index=w260) -> (w261:u16[])
          n147 = call "BRig_RT__Case_Idle__calc_LaserPulse.vi"("input_dataExp_L_Tshutter"=w255, "input_dataExp_L_Tpeak"=w256, "input_dataExp_L_T"=w258, "input_dataExp_L_freq"=w257, "input_dataExp"=w264) -> ("output_cluster"=→"LaserPulseTrain":cluster{u16[], u16[]})  [unwired: 6 in]
        }
      }
    }
    frame True {
      w301 = 100.0 ("y")
      n148 = call "BRig_dataLC_ENL_First_OnOff_l1.vi"() -> ("output_ENL_First_OnOff"=w443:i32)  [unwired: 11 in]
      n149 = call "BRig_dataLC_ENL_First_Block_l1.vi"() -> ("output_ENL_First_Block"=w442:i32)  [unwired: 11 in]
      n150 = call "BRig_dataLC_ENL_First_Prob_l1.vi"() -> ("output_ENL_First_Prob"=w441:i32)  [unwired: 11 in]
      n151 = call "BRig_dataLC_ENL_First_Delay_l1.vi"() -> ("output_ENL_First_Delay"=w440:i32)  [unwired: 11 in]
      n152 = call "BRig_dataLC_ENL_First_DelayOpt_l1.vi"() -> ("output_ENL_First_DelayOpt"=w439:i32)  [unwired: 11 in]
      n153 = call "BRig_dataLC_ENL_First_Count_l1.vi"() -> ("output_ENL_First_Count"=w438:i32)  [unwired: 11 in]
      n154 = call "BRig_dataLC_ENL_PreR_OnOff_l1.vi"() -> ("output_ENL_PreR_OnOff"=w437:i32)  [unwired: 11 in]
      n155 = call "BRig_dataLC_ENL_PreR_Block_l1.vi"() -> ("output_ENL_PreR_Block"=w436:i32)  [unwired: 11 in]
      n156 = call "BRig_dataLC_ENL_PreR_Prob_l1.vi"() -> ("output_ENL_PreR_Prob"=w435:i32)  [unwired: 11 in]
      n157 = call "BRig_dataLC_ENL_PreR_Delay_l1.vi"() -> ("output_ENL_PreR_Delay"=w434:i32)  [unwired: 11 in]
      n158 = call "BRig_dataLC_ENL_PreR_DelayOpt_l1.vi"() -> ("output_ENL_PreR_DelayOpt"=w433:i32)  [unwired: 11 in]
      n159 = call "BRig_dataLC_ENL_PreR_Count_l1.vi"() -> ("output_ENL_PreR_Count"=w432:i32)  [unwired: 11 in]
      n160 = call "BRig_dataLC_ENL_PostR_OnOff_l1.vi"() -> ("output_ENL_PostR_OnOff"=w431:i32)  [unwired: 11 in]
      n161 = call "BRig_dataLC_ENL_PostR_Block_l1.vi"() -> ("output_ENL_PostR_Block"=w430:i32)  [unwired: 11 in]
      n162 = call "BRig_dataLC_ENL_PostR_Prob_l1.vi"() -> ("output_ENL_PostR_Prob"=w429:i32)  [unwired: 11 in]
      n163 = call "BRig_dataLC_ENL_PostR_Delay_l1.vi"() -> ("output_ENL_PostR_Delay"=w428:i32)  [unwired: 11 in]
      n164 = call "BRig_dataLC_ENL_PostR_DelayOpt_l1.vi"() -> ("output_ENL_PostR_DelayOpt"=w427:i32)  [unwired: 11 in]
      n165 = call "BRig_dataLC_ENL_PostR_Count_l1.vi"() -> ("output_ENL_PostR_Count"=w426:i32)  [unwired: 11 in]
      n166 = call "BRig_dataLC_Reward_nRew1_l1.vi"() -> ("output_Reward_nRew1_l1"=w280:i32)  [unwired: 11 in]
      n167 = call "BRig_dataLC_Reward_nRew2_l1.vi"() -> ("output_Reward_nRew2_l1"=w279:i32)  [unwired: 11 in]
      n168 = call "BRig_dataLC_Wrong_nRew1_l1.vi"() -> ("output_Wrong_nRew1_l1"=w276:i32)  [unwired: 11 in]
      n169 = call "BRig_dataLC_Wrong_nRew2_l1.vi"() -> ("output_Wrong_nRew2_l1"=w275:i32)  [unwired: 11 in]
      n170 = Index Array(array=w281, index #1=w280, index #2=w279, index #3=w276, index #4=w275) -> (element #1=w278:u16, element #2=w277:u16, element #3=w274:u16, element #4=w273:u16)
      n171 = Index Array(array=w281, index #1=w443, index #2=w442, index #3=w441, index #4=w440, index #5=w439, index #6=w438, index #7=w437, index #8=w436, index #9=w435, index #10=w434, index #11=w433, index #12=w432, index #13=w431, index #14=w430, index #15=w429, index #16=w428, index #17=w427, index #18=w426) -> (element #1=w419:u16, element #2=w418:u16, element #3=w417:u16, element #4=w416:u16, element #5=w415:u16, element #6=w414:u16, element #7=w413:u16, element #8=w412:u16, element #9=w411:u16, element #10=w410:u16, element #11=w409:u16, element #12=w408:u16, element #13=w407:u16, element #14=w406:u16, element #15=w405:u16, element #16=w404:u16, element #17=w403:u16, element #18=w402:u16)
      n172 = local write "LC_Rew_nRew1"(w278) -> ()
      n173 = local write "LC_Rew_nRew2"(w277) -> ()
      n174 = local write "LC_Wro_nRew1"(w274) -> ()
      n175 = local write "LC_Wro_nRew2"(w273) -> ()
      n176 = Not Equal To 0?(x=w419) -> (x != 0?=w425:bool)
      n177 = Not Equal To 0?(x=w415) -> (x != 0?=w424:bool)
      n178 = Not Equal To 0?(x=w413) -> (x != 0?=w423:bool)
      n179 = Not Equal To 0?(x=w409) -> (x != 0?=w422:bool)
      n180 = Not Equal To 0?(x=w407) -> (x != 0?=w421:bool)
      n181 = Not Equal To 0?(x=w403) -> (x != 0?=w420:bool)
      n182 = local write "LC_ENL_First_OnOff"(w425) -> ()
      n183 = local write "LC_ENL_First_Block"(w418) -> ()
      n184 = local write "LC_ENL_First_Probability"(w417) -> ()
      n185 = local write "LC_ENL_First_Tdelay"(w416) -> ()
      n186 = local write "LC_ENL_First_delayOpt"(w424) -> ()
      n187 = local write "LC_ENL_First_Count"(w414) -> ()
      n188 = local write "LC_ENL_PreR_OnOff"(w423) -> ()
      n189 = local write "LC_ENL_PreR_Block"(w412) -> ()
      n190 = local write "LC_ENL_PreR_Probability"(w411) -> ()
      n191 = local write "LC_ENL_PreR_Tdelay"(w410) -> ()
      n192 = local write "LC_ENL_PreR_delayOpt"(w422) -> ()
      n193 = local write "LC_ENL_PreR_Count"(w408) -> ()
      n194 = local write "LC_ENL_PostR_OnOff"(w421) -> ()
      n195 = local write "LC_ENL_PostR_Block"(w406) -> ()
      n196 = local write "LC_ENL_PostR_Probability"(w405) -> ()
      n197 = local write "LC_ENL_PostR_Tdelay"(w404) -> ()
      n198 = local write "LC_ENL_PostR_delayOpt"(w420) -> ()
      n199 = local write "LC_ENL_PostR_Count"(w402) -> ()
      n200 = call "BRig_dataLC_Cue_PreR_OnOff_l1.vi"() -> ("output_Cue_PreR_OnOff"=w291:i32)  [unwired: 11 in]
      n201 = call "BRig_dataLC_Cue_PreR_Block_l1.vi"() -> ("output_Cue_PreR_Block"=w290:i32)  [unwired: 11 in]
      n202 = call "BRig_dataLC_Cue_PreR_Prob_l1.vi"() -> ("output_Cue_PreR_Prob"=w289:i32)  [unwired: 11 in]
      n203 = call "BRig_dataLC_Cue_PreR_Delay_l1.vi"() -> ("output_Cue_PreR_Delay"=w288:i32)  [unwired: 11 in]
      n204 = call "BRig_dataLC_Cue_PreR_DelayOpt_l1.vi"() -> ("output_Cue_PreR_DelayOpt"=w287:i32)  [unwired: 11 in]
      n205 = call "BRig_dataLC_Cue_PreR_Count_l1.vi"() -> ("output_Cue_PreR_Count"=w292:i32)  [unwired: 11 in]
      n206 = call "BRig_dataLC_Cue_First_OnOff_l1.vi"() -> ("output_Cue_First_OnOff"=w449:i32)  [unwired: 11 in]
      n207 = call "BRig_dataLC_Cue_First_Block_l1.vi"() -> ("output_Cue_First_Block"=w448:i32)  [unwired: 11 in]
      n208 = call "BRig_dataLC_Cue_First_Prob_l1.vi"() -> ("output_Cue_First_Prob"=w447:i32)  [unwired: 11 in]
      n209 = call "BRig_dataLC_Cue_First_Delay_l1.vi"() -> ("output_Cue_First_Delay"=w446:i32)  [unwired: 11 in]
      n210 = call "BRig_dataLC_Cue_First_DelayOpt_l1.vi"() -> ("output_Cue_First_DelayOpt"=w445:i32)  [unwired: 11 in]
      n211 = call "BRig_dataLC_Cue_First_Count_l1.vi"() -> ("output_Cue_First_Count"=w444:i32)  [unwired: 11 in]
      n212 = call "BRig_dataLC_Cue_PostR_OnOff_l1.vi"() -> ("output_Cue_PostR_OnOff"=w297:i32)  [unwired: 11 in]
      n213 = call "BRig_dataLC_Cue_PostR_Block_l1.vi"() -> ("output_Cue_PostR_Block"=w296:i32)  [unwired: 11 in]
      n214 = call "BRig_dataLC_Cue_PostR_Prob_l1.vi"() -> ("output_Cue_PostR_Prob"=w295:i32)  [unwired: 11 in]
      n215 = call "BRig_dataLC_Cue_PostR_Delay_l1.vi"() -> ("output_Cue_PostR_Delay"=w294:i32)  [unwired: 11 in]
      n216 = call "BRig_dataLC_Cue_PostR_DelayOpt_l1.vi"() -> ("output_Cue_PostR_DelayOpt"=w293:i32)  [unwired: 11 in]
      n217 = call "BRig_dataLC_Cue_PostR_Count_l1.vi"() -> ("output_Cue_PostR_Count"=w298:i32)  [unwired: 11 in]
      n218 = call "BRig_dataExp_LED_baseline_Cue.vi"() -> ("output_LED_baseline_Cue"=w322:i32)  [unwired: 11 in]
      n219 = call "BRig_dataExp_L_freq_l1.vi"() -> ("output_L_freq_l1"=w321:i32)  [unwired: 11 in]
      n220 = call "BRig_dataExp_L_T_l1.vi"() -> ("output_L_T_l1"=w320:i32)  [unwired: 11 in]
      n221 = call "BRig_dataExp_L_Tpeak_l1.vi"() -> ("output_L_Tpeak_l1"=w319:i32)  [unwired: 11 in]
      n222 = call "BRig_dataExp_L_Tshutter_l1.vi"() -> ("output_L_Tshutter_l1"=w318:i32)  [unwired: 11 in]
      n223 = call "BRig_dataExp_L_power_min_l1.vi"() -> ("output_L_power_min_l1"=w317:i32)  [unwired: 11 in]
      n224 = call "BRig_dataExp_L_power_max_l1.vi"() -> ("output_L_power_max_l1"=w316:i32)  [unwired: 11 in]
      n225 = call "BRig_dataExp_L_power_step_l1.vi"() -> ("output_L_power_step_l1"=w315:i32)  [unwired: 11 in]
      n226 = Index Array(array=w281, index #1=w449, index #2=w448, index #3=w447, index #4=w446, index #5=w445, index #6=w444, index #7=w291, index #8=w290, index #9=w289, index #10=w288, index #11=w287, index #12=w292, index #13=w297, index #14=w296, index #15=w295, index #16=w294, index #17=w293, index #18=w298) -> (element #1=w395:u16, element #2=w394:u16, element #3=w393:u16, element #4=w392:u16, element #5=w391:u16, element #6=w390:u16, element #7=w389:u16, element #8=w388:u16, element #9=w387:u16, element #10=w386:u16, element #11=w385:u16, element #12=w384:u16, element #13=w383:u16, element #14=w382:u16, element #15=w381:u16, element #16=w380:u16, element #17=w379:u16, element #18=w378:u16)
      n227 = Index Array(array=w282, index #1=w322, index #2=w321, index #3=w320, index #4=w319, index #5=w318, index #6=w317, index #7=w316, index #8=w315) -> (element #1=w314:u16, element #2=w312:u16, element #3=w311:u16, element #4=w310:u16, element #5=w309:u16, element #6=w308:u16, element #7=w307:u16, element #8=w306:u16)
      n228 = To Double Precision Float(number=w308) -> (double precision float=w305:dbl)
      n229 = To Double Precision Float(number=w307) -> (double precision float=w300:dbl)
      n230 = To Double Precision Float(number=w306) -> (double precision float=w299:dbl)
      n231 = Not Equal To 0?(x=w395) -> (x != 0?=w401:bool)
      n232 = Not Equal To 0?(x=w391) -> (x != 0?=w400:bool)
      n233 = Not Equal To 0?(x=w389) -> (x != 0?=w399:bool)
      n234 = Not Equal To 0?(x=w385) -> (x != 0?=w398:bool)
      n235 = Not Equal To 0?(x=w383) -> (x != 0?=w397:bool)
      n236 = Not Equal To 0?(x=w379) -> (x != 0?=w396:bool)
      n237 = Divide(x=w305, y=w301) -> (x/y=w304:dbl)
      n238 = Divide(x=w300, y=w301) -> (x/y=w303:dbl)
      n239 = Divide(x=w299, y=w301) -> (x/y=w302:dbl)
      n240 = local write "LC_Cue_First_OnOff"(w401) -> ()
      n241 = local write "LC_Cue_First_Block"(w394) -> ()
      n242 = local write "LC_Cue_First_Probability"(w393) -> ()
      n243 = local write "LC_Cue_First_Tdelay"(w392) -> ()
      n244 = local write "LC_Cue_First_delayOpt"(w400) -> ()
      n245 = local write "LC_Cue_First_Count"(w390) -> ()
      n246 = local write "LC_Cue_PreR_OnOff"(w399) -> ()
      n247 = local write "LC_Cue_PreR_Block"(w388) -> ()
      n248 = local write "LC_Cue_PreR_Probability"(w387) -> ()
      n249 = local write "LC_Cue_PreR_Tdelay"(w386) -> ()
      n250 = local write "LC_Cue_PreR_delayOpt"(w398) -> ()
      n251 = local write "LC_Cue_PreR_Count"(w384) -> ()
      n252 = local write "LC_Cue_PostR_OnOff"(w397) -> ()
      n253 = local write "LC_Cue_PostR_Block"(w382) -> ()
      n254 = local write "LC_Cue_PostR_Probability"(w381) -> ()
      n255 = local write "LC_Cue_PostR_Tdelay"(w380) -> ()
      n256 = local write "LC_Cue_PostR_delayOpt"(w396) -> ()
      n257 = local write "LC_Cue_PostR_Count"(w378) -> ()
      n258 = Not Equal To 0?(x=w314) -> (x != 0?=w313:bool)
      n259 = local write "LED_baseline"(w313) -> ()
      n260 = local write "Laser_Freq"(w312) -> ()
      n261 = local write "Laser_T"(w311) -> ()
      n262 = local write "Laser_Tpeak"(w310) -> ()
      n263 = local write "Laser_Tshutter"(w309) -> ()
      n264 = local write "Laser_power_min"(w304) -> ()
      n265 = local write "Laser_power_max"(w303) -> ()
      n266 = local write "Laser_power_step"(w302) -> ()
      n267 = call "BRig_dataLC_Selection_PostR_OnOff_l1.vi"() -> ("output_Selection_PostR_OnOff"=w367:i32)  [unwired: 11 in]
      n268 = call "BRig_dataLC_Selection_PostR_Block_l1.vi"() -> ("output_Selection_PostR_Block"=w366:i32)  [unwired: 11 in]
      n269 = call "BRig_dataLC_Selection_PostR_Prob_l1.vi"() -> ("output_Selection_PostR_Prob"=w365:i32)  [unwired: 11 in]
      n270 = call "BRig_dataLC_Selection_PostR_Delay_l1.vi"() -> ("output_Selection_PostR_Delay"=w364:i32)  [unwired: 11 in]
      n271 = call "BRig_dataLC_Selection_PostR_Count_l1.vi"() -> ("output_Selection_PostR_Count"=w363:i32)  [unwired: 11 in]
      n272 = call "BRig_dataLC_Selection_PreR_OnOff_l1.vi"() -> ("output_Selection_PreR_OnOff"=w372:i32)  [unwired: 11 in]
      n273 = call "BRig_dataLC_Selection_PreR_Block_l1.vi"() -> ("output_Selection_PreR_Block"=w371:i32)  [unwired: 11 in]
      n274 = call "BRig_dataLC_Selection_PreR_Prob_l1.vi"() -> ("output_Selection_PreR_Prob"=w370:i32)  [unwired: 11 in]
      n275 = call "BRig_dataLC_Selection_PreR_Delay_l1.vi"() -> ("output_Selection_PreR_Delay"=w369:i32)  [unwired: 11 in]
      n276 = call "BRig_dataLC_Selection_PreR_Count_l1.vi"() -> ("output_Selection_PreR_Count"=w368:i32)  [unwired: 11 in]
      n277 = call "BRig_dataLC_Selection_First_OnOff_l1.vi"() -> ("output_Selection_First_OnOff"=w377:i32)  [unwired: 11 in]
      n278 = call "BRig_dataLC_Selection_First_Block_l1.vi"() -> ("output_Selection_First_Block"=w376:i32)  [unwired: 11 in]
      n279 = call "BRig_dataLC_Selection_First_Prob_l1.vi"() -> ("output_Selection_First_Prob"=w375:i32)  [unwired: 11 in]
      n280 = call "BRig_dataLC_Selection_First_Delay_l1.vi"() -> ("output_Selection_First_Delay"=w374:i32)  [unwired: 11 in]
      n281 = call "BRig_dataLC_Selection_First_Count_l1.vi"() -> ("output_Selection_First_Count"=w373:i32)  [unwired: 11 in]
      n282 = call "BRig_dataLC_Reward_OnOff_l1.vi"() -> ("output_Reward_OnOff"=w344:i32)  [unwired: 11 in]
      n283 = call "BRig_dataLC_Reward_Block_l1.vi"() -> ("output_Reward_Block"=w343:i32)  [unwired: 11 in]
      n284 = call "BRig_dataLC_Reward_Trial_l1.vi"() -> ("output_Reward_Trial"=w342:i32)  [unwired: 11 in]
      n285 = call "BRig_dataLC_Reward_Prob_l1.vi"() -> ("output_Reward_Prob"=w341:i32)  [unwired: 11 in]
      n286 = call "BRig_dataLC_Reward_Delay_l1.vi"() -> ("output_Reward_Delay"=w340:i32)  [unwired: 11 in]
      n287 = call "BRig_dataLC_Wrong_OnOff_l1.vi"() -> ("output_Wrong_OnOff"=w339:i32)  [unwired: 11 in]
      n288 = call "BRig_dataLC_Wrong_Block_l1.vi"() -> ("output_Wrong_Block"=w338:i32)  [unwired: 11 in]
      n289 = call "BRig_dataLC_Wrong_Trial_l1.vi"() -> ("output_Wrong_Trial"=w337:i32)  [unwired: 11 in]
      n290 = call "BRig_dataLC_Wrong_Prob_l1.vi"() -> ("output_Wrong_Prob"=w336:i32)  [unwired: 11 in]
      n291 = call "BRig_dataLC_Wrong_Delay_l1.vi"() -> ("output_Wrong_Delay"=w335:i32)  [unwired: 11 in]
      n292 = call "BRig_dataLC_ENL_PostR_nRew1_l1.vi"() -> ("output_ENL_PostR_nRew1_l1"=w286:i32)  [unwired: 11 in]
      n293 = call "BRig_dataLC_ENL_PostR_nRew2_l1.vi"() -> ("output_ENL_PostR_nRew2_l1"=w285:i32)  [unwired: 11 in]
      n294 = call "BRig_dataLC_Cue_PostR_nRew1_l1.vi"() -> ("output_Cue_PostR_nRew1_l1"=w272:i32)  [unwired: 11 in]
      n295 = call "BRig_dataLC_Cue_PostR_nRew2_l1.vi"() -> ("output_Cue_PostR_nRew2_l1"=w271:i32)  [unwired: 11 in]
      n296 = call "BRig_dataLC_Selection_PostR_nRew1_l1.vi"() -> ("output_Selection_PostR_nRew1_l1"=w268:i32)  [unwired: 11 in]
      n297 = call "BRig_dataLC_Selection_PostR_nRew2_l1.vi"() -> ("output_Selection_PostR_nRew2_l1"=w267:i32)  [unwired: 11 in]
      n298 = Index Array(array=w281, index #1=w344, index #2=w343, index #3=w342, index #4=w341, index #5=w340, index #6=w339, index #7=w338, index #8=w337, index #9=w336, index #10=w335) -> (element #1=w332:u16, element #2=w331:u16, element #3=w330:u16, element #4=w329:u16, element #5=w328:u16, element #6=w327:u16, element #7=w326:u16, element #8=w325:u16, element #9=w324:u16, element #10=w323:u16)
      n299 = Index Array(array=w281, index #1=w377, index #2=w376, index #3=w375, index #4=w374, index #5=w373, index #6=w372, index #7=w371, index #8=w370, index #9=w369, index #10=w368, index #11=w367, index #12=w366, index #13=w365, index #14=w364, index #15=w363) -> (element #1=w359:u16, element #2=w358:u16, element #3=w357:u16, element #4=w356:u16, element #5=w355:u16, element #6=w354:u16, element #7=w353:u16, element #8=w352:u16, element #9=w351:u16, element #10=w350:u16, element #11=w349:u16, element #12=w348:u16, element #13=w347:u16, element #14=w346:u16, element #15=w345:u16)
      n300 = Not Equal To 0?(x=w332) -> (x != 0?=w334:bool)
      n301 = Not Equal To 0?(x=w327) -> (x != 0?=w333:bool)
      n302 = Not Equal To 0?(x=w359) -> (x != 0?=w362:bool)
      n303 = Not Equal To 0?(x=w354) -> (x != 0?=w361:bool)
      n304 = Not Equal To 0?(x=w349) -> (x != 0?=w360:bool)
      n305 = Index Array(array=w281, index #1=w286, index #2=w285, index #3=w272, index #4=w271, index #5=w268, index #6=w267) -> (element #1=w284:u16, element #2=w283:u16, element #3=w270:u16, element #4=w269:u16, element #5=w266:u16, element #6=w265:u16)  [unwired: 4 in, 4 out]
      n306 = local write "LC_Reward_OnOff"(w334) -> ()
      n307 = local write "LC_Reward_Block"(w331) -> ()
      n308 = local write "LC_Reward_Trial"(w330) -> ()
      n309 = local write "LC_Reward_Probability"(w329) -> ()
      n310 = local write "LC_Reward_Tdelay"(w328) -> ()
      n311 = local write "LC_Wrong_OnOff"(w333) -> ()
      n312 = local write "LC_Wrong_Block"(w326) -> ()
      n313 = local write "LC_Wrong_Trial"(w325) -> ()
      n314 = local write "LC_Wrong_Probability"(w324) -> ()
      n315 = local write "LC_Wrong_Tdelay"(w323) -> ()
      n316 = local write "LC_Sel_First_OnOff"(w362) -> ()
      n317 = local write "LC_Sel_First_Block"(w358) -> ()
      n318 = local write "LC_Sel_First_Probability"(w357) -> ()
      n319 = local write "LC_Sel_First_Tdelay"(w356) -> ()
      n320 = local write "LC_Sel_First_Count"(w355) -> ()
      n321 = local write "LC_Sel_PreR_OnOff"(w361) -> ()
      n322 = local write "LC_Sel_PreR_Block"(w353) -> ()
      n323 = local write "LC_Sel_PreR_Probability"(w352) -> ()
      n324 = local write "LC_Sel_PreR_Tdelay"(w351) -> ()
      n325 = local write "LC_Sel_PreR_Count"(w350) -> ()
      n326 = local write "LC_Sel_PostR_OnOff"(w360) -> ()
      n327 = local write "LC_Sel_PostR_Block"(w348) -> ()
      n328 = local write "LC_Sel_PostR_Probability"(w347) -> ()
      n329 = local write "LC_Sel_PostR_Tdelay"(w346) -> ()
      n330 = local write "LC_Sel_PostR_Count"(w345) -> ()
      n331 = local write "LC_ENL_nRew1"(w284) -> ()
      n332 = local write "LC_ENL_nRew2"(w283) -> ()
      n333 = local write "LC_Cue_nRew1"(w270) -> ()
      n334 = local write "LC_Cue_nRew2"(w269) -> ()
      n335 = local write "LC_Sel_nRew1"(w266) -> ()
      n336 = local write "LC_Sel_nRew2"(w265) -> ()
    }
  }
  "output_dataLC" <- w4
  "output_dataExp" <- w1
